vi "onAssertionSlippage.vi"(7 "AssertFalse in":refnum<class "AssertFalse.lvclass">, 10 "Properties":refnum<class "Properties.Assert.lvclass">) -> (0 "error out":errorcluster, 2 "Properties out":refnum<class "Properties.Assert.lvclass">)   [LabVIEW 2021, in "Bananas.lvlib" / "AssertFalse.lvclass"]
uses:
  AssertFalse.lvclass
  AssertFalse.lvclass/AssertFalse.ctl
  <vilib>/addons/_JKI Toolkits/Caraya/classes/Properties.Assert/Properties.Assert.lvclass
  <vilib>/addons/_JKI Toolkits/Caraya/classes/Properties/Properties.lvclass
  C:/Program Files (x86)/National Instruments/LabVIEW 2021/vi.lib/addons/_JKI Toolkits/Caraya/classes/Properties/Properties.lvclass
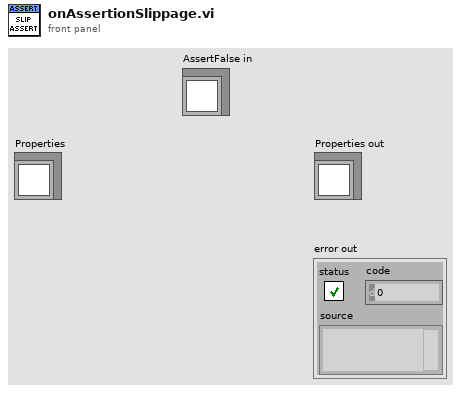
[diagram p1: front panel]
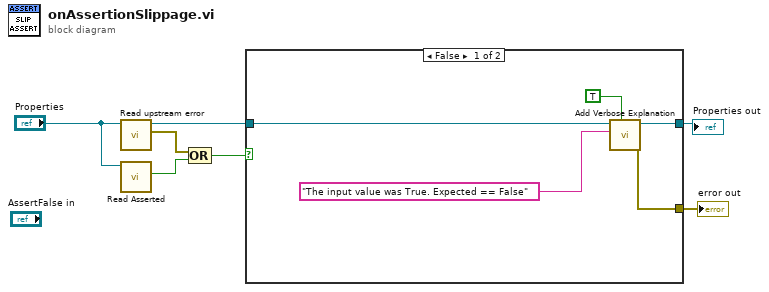
[diagram p0: block diagram]
diagram:
  n1 = call <vilib>:"Read upstream error.vi"("Properties.Assert in"="Properties") -> ("upstream-error"=w6:errorcluster, "Properties.Assert out"=w7:refnum<class "Properties.Assert.lvclass">)  [unwired: 9 in]
  n2 = call <vilib>:"Read Asserted.vi"("Properties.Assert in"="Properties") -> ("Asserted"=w5:bool)  [unwired: 9 in, 1 out]
  n3 = Compound Arithmetic op=OR(w6, w5) -> (w4:bool)
  n4 = case shown="False" w4 {
    tunnel: [w11 w13] -> w2
    tunnel: [w10 _] -> w1
    tunnel: w7 -> [w12 w13]
    frame False {
      n5 = call <vilib>:"Add Verbose Explanation.vi"("overwrite?"=TRUE, "Verbose Explanation"="The input value was True. Expected == False", "Properties"=w12) -> ("error out"=w10:errorcluster, "Properties"=w11:refnum<class "Properties.Assert.lvclass">)  [unwired: 7 in]
    }
    frame True {
      # "There was an upstream error or the assertion = TRUE"
    }
  }
  "error out" <- w1
  "Properties out" <- w2
